vi "quadratic-roots.vi"() -> ()   [LabVIEW 2025]
panel:
  out "Root 2":dbl
  out "Root 1":dbl
  in  "C":dbl
  in  "B":dbl
  in  "A":dbl
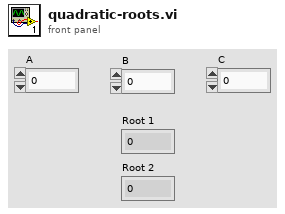
[diagram p1: front panel]
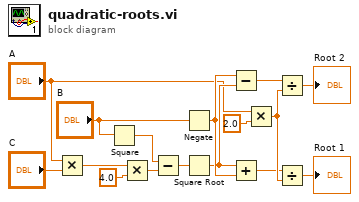
[diagram p0: block diagram]
diagram:
  n1 = Multiply(x="A", y="C") -> (x*y=w15:dbl)
  n2 = Square(x="B") -> (x^2=w13:dbl)
  n3 = Multiply(x=w15, y=4.0) -> (x*y=w12:dbl)
  n4 = Subtract(x=w13, y=w12) -> (x-y=w11:dbl)
  n5 = Negate(x="B") -> (-x=w9:dbl)
  n6 = Square Root(x=w11) -> (sqrt(x)=w8:dbl)
  n7 = Subtract(x=w9, y=w8) -> (x-y=w5:dbl)
  n8 = Add(x=w8, y=w9) -> (x+y=w3:dbl)
  n9 = Multiply(x="A", y=2.0) -> (x*y=w4:dbl)
  n10 = Divide(x=w5, y=w4) -> (x/y=→"Root 2":dbl)
  n11 = Divide(x=w3, y=w4) -> (x/y=→"Root 1":dbl)
